vi "GetText.vi"(8 "error in":errorcluster, 11 "node in":refnum<class "My System.lvclass">) -> (0 "error out":errorcluster, 1 "additional text":string, 2 "text":string, 3 "node out":refnum<class "My System.lvclass">, 4 "glyph":string)   [LabVIEW 2014, in "My System.lvclass"]
doc: "Returns the text representation of the node used for the tree control."
uses:
  My System.lvclass
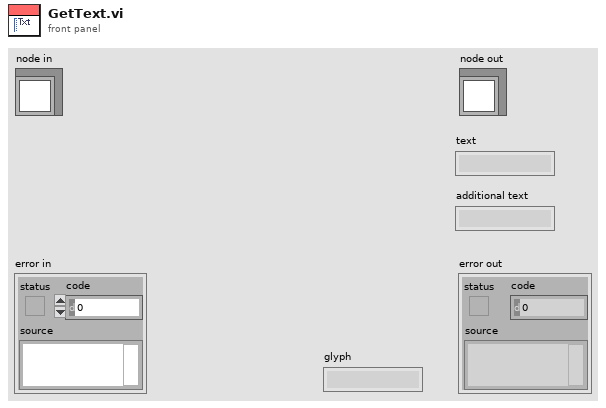
[diagram p1: front panel]
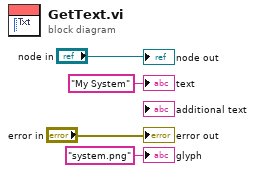
[diagram p0: block diagram]
diagram:
  "error out" <- "error in"
  "node out" <- "node in"
  "text" <- "My System" ("text")
  "glyph" <- "system.png" ("glyph")
